vi "Serialize and Deserialize Configuration.vi"() -> ()   [LabVIEW 2013]
uses:
  <vilib>/Utility/xml.llb/Write to XML File(array).vi
  <vilib>/xml/Load XML File.vi
  <vilib>/xml/NI_XML.lvlib
panel:
  in  "Load":bool
  in  "Save":bool
  in  "XML File Path":path
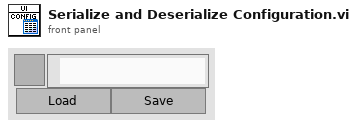
[diagram p1: front panel]
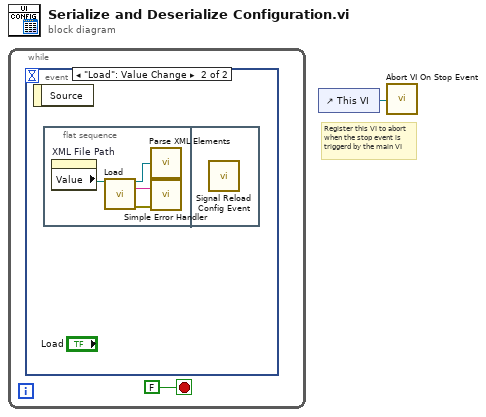
[diagram p0: block diagram]
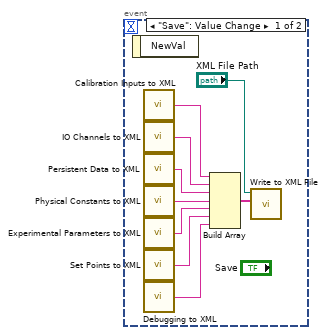
[diagram p2: hidden frame]
diagram:
  # "Register this VI to abort\nwhen the stop event is\ntriggerd by the main VI"
  n1 = while {
    stop <- FALSE stop-if-true
    n2 = event shown="[1] \"Load\": Value Change" {
      selector: _ -> [_ _]
      dyn-events: _ -> [_ _]
      timeout: _ -> [_ _]
      event "Save": Value Change {
        n3 = event-data() -> ()  [unwired: 1 in, 1 out]
        n4 = call "Calibration Inputs to XML.vi"() -> ("XML Data"=w5:string)
        n5 = call "IO Channels to XML.vi"() -> ("XML Data"=w6:string)
        n6 = call "Persistent Data to XML.vi"() -> ("XML Data"=w10:string)
        n7 = call "Physical Constants to XML.vi"() -> ("XML Data"=w11:string)
        n8 = call "Experimental Parameters to XML.vi"() -> ("XML Data"=w9:string)
        n9 = call "Set Points to XML.vi"() -> ("XML Data"=w8:string)
        n10 = call "Debugging to XML.vi"() -> ("XML Data"=w7:string)
        n11 = Build Array(w5, w6, w10, w11, w9, w8, w7) -> (w4:string[])
        n12 = call-poly <vilib>:"Write to XML File.vi"("XML Input"=w4, "XML File Path"="XML File Path") -> ()  [unwired: 7 in, 3 out]
      }
      event "Load": Value Change {
        n13 = event-data() -> ()  [unwired: 1 in, 1 out]
        n14 = flat-sequence {
          frame #0 {
            n15 = property on="XML File Path" class="Path"() -> ("Value"=w13:path)  [unwired: 2 in, 2 out]
            n16 = call-poly <vilib>:"Load.vi"("path to XML document"=w13) -> ("DOM document out"=w12:refnum<k20>, "parse errors"=w15:string, "error out"=w14:errorcluster)  [unwired: 12 in]
            n17 = call "Parse XML Elements.vi"("DOM"=w12) -> ()
            n18 = call <vilib>:"Simple Error Handler.vi"("error source (\" \")"=w15, "error in (no error)"=w14) -> ()  [unwired: 3 in, 5 out]
          }
          frame #1 {
            n19 = call "Signal Reload Config Event.vi"() -> ()  [unwired: 1 in]
          }
        }
      }
    }
  }
  n20 = control-ref of="This VI"() -> (w1:refnum<vi>)
  n21 = call "Abort VI On Stop Event.vi"("VI Reference"=w1) -> ()
